vi "XCursorSlider.vi"(0 "IntensityGraph in":refnum<vi>, 1 "Cursor\nHold-off":dbl, 2 "Distance betweed scan lines (um)":sgl, 3 "Force Symmetric?":bool=TRUE) -> (4 "Scan Size X (mm)":dbl, 5 "lines per plane":i32, 6 "Scan Center (mm)":dbl)   [LabVIEW 2022 SP3]
uses:
  <vilib>/Analysis/baseanly.llb/Mean (DBL).vi
  Misc Programs/MathOperations/ModuloFraction.vi
  <vilib>/Analysis/NI_AALBase.lvlib
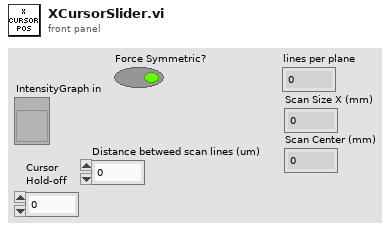
[diagram p1: front panel]
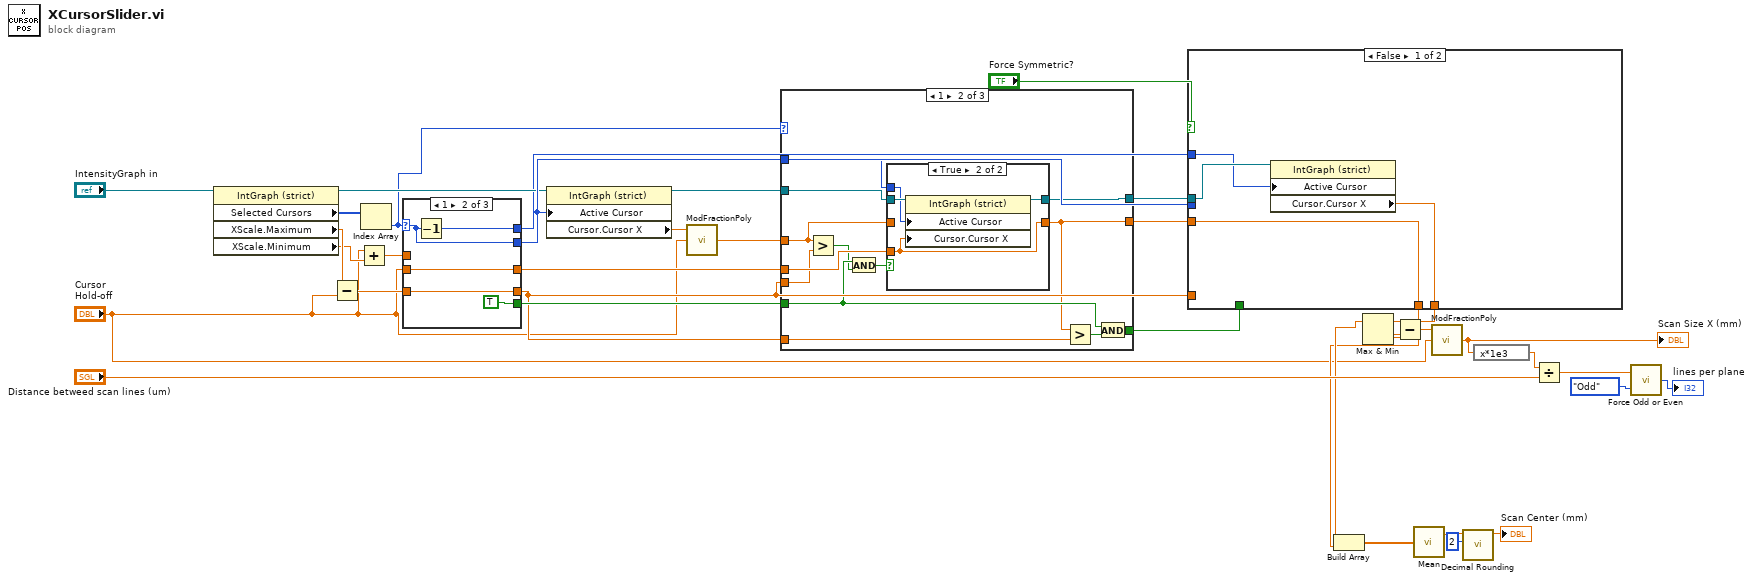
[diagram p0: block diagram]
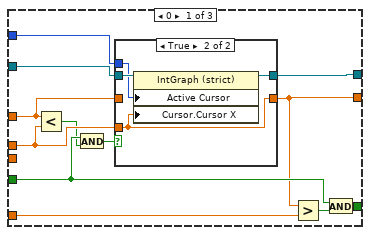
[diagram p2: hidden frame]
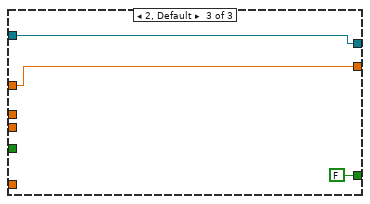
[diagram p5: hidden frame]
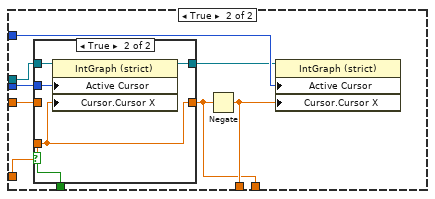
[diagram p6: hidden frame]
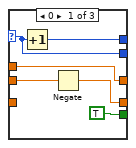
[diagram p8: hidden frame]
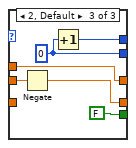
[diagram p9: hidden frame]
diagram:
  n1 = property class="IntGraph (strict)"(reference="IntensityGraph in") -> (reference out=w27:refnum<vi>, "Selected Cursors"=w25:u32[], "XScale.Maximum"=w17:dbl, "XScale.Minimum"=w16:dbl)  [unwired: 1 in, 1 out]
  n2 = Subtract(x=w17, y="Cursor\nHold-off") -> (x-y=w2:dbl)
  n3 = Add(x="Cursor\nHold-off", y=w16) -> (x+y=w29:dbl)
  n4 = Index Array(array=w25) -> (element=w4:u32)  [unwired: 1 in]
  n5 = case shown="1" w4 {
    selector: w4 -> [w38 w44 _]
    tunnel: [w38 w44 w53] -> w34
    tunnel: [TRUE TRUE FALSE] -> w33
    tunnel: [w37 w43 w51] -> w23
    tunnel: [w41 w45 w50] -> w30
    tunnel: w29 -> [w41 _ w50]
    tunnel: [w39 w46 w48] -> w3
    tunnel: w2 -> [_ w46 _]
    tunnel: "Cursor\nHold-off" -> [w40 w45 w49]
    frame 0 {
      n6 = Increment(x=w38) -> (x+1=w37:u32)
      n7 = Negate(x=w40) -> (-x=w39:dbl)
    }
    frame 1 {
      n8 = Decrement(x=w44) -> (x-1=w43:u32)
    }
    frame 2, Default {
      w53 = u32 0 ("Active Cursor")
      n9 = Negate(x=w49) -> (-x=w48:dbl)
      n10 = Increment(x=w53) -> (x+1=w51:u32)
    }
  }
  n11 = property on="Property Node" class="IntGraph (strict)"(reference=w27, "Active Cursor"=w34) -> (reference out=w28:refnum<vi>, "Cursor.Cursor X"=w35:dbl)  [unwired: 1 in, 1 out]
  n12 = call-poly "ModFractionPoly.vi"("Modulo Fraction"="Cursor\nHold-off", "Input"=w35) -> ("Output"=w36:dbl)  [unwired: 1 in]
  n13 = case shown="1" w4 {
    tunnel: w36 -> [w65 w84 w92]
    tunnel: w34 -> [w64 w83 _]
    tunnel: w33 -> [w63 w82 _]
    tunnel: [w62 w81 FALSE] -> w32
    tunnel: [w60 w79 w92] -> w31
    tunnel: w3 -> [w59 w78 _]
    tunnel: w30 -> [w58 w77 _]
    tunnel: w28 -> [w57 w76 w93]
    tunnel: [w54 w73 w93] -> w24
    tunnel: w3 -> [_ w72 _]
    frame 0 {
      n14 = Less?(x=w65, y=w58) -> (x < y?=w55:bool)
      n15 = And(x=w63, y=w55) -> (x .and. y?=w61:bool)
      n16 = case shown="True" w61 {
        tunnel: w57 -> [w66 w71]
        tunnel: w58 -> [_ w70]
        tunnel: [w67 w70] -> w60
        tunnel: w65 -> [w67 _]
        tunnel: w64 -> [_ w69]
        tunnel: [w66 w68] -> w54
        frame False {
        }
        frame True {
          n17 = property on="Property Node" class="IntGraph (strict)"(reference=w71, "Active Cursor"=w69, "Cursor.Cursor X"=w70) -> (reference out=w68:refnum<vi>)  [unwired: 1 in, 1 out]
        }
      }
      n18 = Greater?(x=w60, y=w59) -> (0:w56:bool)
      n19 = And(x=w63, y=w56) -> (x .and. y?=w62:bool)
    }
    frame 1 {
      n20 = Greater?(x=w84, y=w72) -> (0:w74:bool)
      n21 = And(x=w82, y=w74) -> (x .and. y?=w80:bool)
      n22 = case shown="True" w80 {
        tunnel: w76 -> [w85 w90]
        tunnel: w77 -> [_ w89]
        tunnel: [w86 w89] -> w79
        tunnel: w84 -> [w86 _]
        tunnel: w83 -> [_ w88]
        tunnel: [w85 w87] -> w73
        frame False {
        }
        frame True {
          n23 = property on="Property Node" class="IntGraph (strict)"(reference=w90, "Active Cursor"=w88, "Cursor.Cursor X"=w89) -> (reference out=w87:refnum<vi>)  [unwired: 1 in, 1 out]
        }
      }
      n24 = Greater?(x=w79, y=w78) -> (0:w75:bool)
      n25 = And(x=w82, y=w75) -> (x .and. y?=w81:bool)
    }
    frame 2, Default {
    }
  }
  n26 = case shown="False" "Force Symmetric?" {
    tunnel: w34 -> [_ w106]
    tunnel: w32 -> [_ w105]
    tunnel: w31 -> [w97 w104]
    tunnel: w3 -> [_ w103]
    tunnel: w24 -> [w96 w102]
    tunnel: w23 -> [w94 w101]
    tunnel: [w97 w100] -> w5
    tunnel: [w95 w98] -> w6
    frame False {
      n27 = property on="Property Node" class="IntGraph (strict)"(reference=w96, "Active Cursor"=w94) -> ("Cursor.Cursor X"=w95:dbl)  [unwired: 1 in, 2 out]
    }
    frame True {
      n28 = case shown="True" w105 {
        tunnel: w103 -> [_ w111]
        tunnel: w102 -> [w107 w112]
        tunnel: [w108 w111] -> w98
        tunnel: w104 -> [w108 _]
        tunnel: w106 -> [_ w110]
        tunnel: [w107 w109] -> w99
        frame False {
        }
        frame True {
          n29 = property on="Property Node" class="IntGraph (strict)"(reference=w112, "Active Cursor"=w110, "Cursor.Cursor X"=w111) -> (reference out=w109:refnum<vi>)  [unwired: 1 in, 1 out]
        }
      }
      n30 = Negate(x=w98) -> (-x=w100:dbl)
      n31 = property on="Property Node" class="IntGraph (strict)"(reference=w99, "Active Cursor"=w101, "Cursor.Cursor X"=w100) -> ()  [unwired: 1 in, 2 out]
    }
  }
  n32 = Build Array(w6, w5) -> (w12:dbl[])
  n33 = Max & Min(x=w6, y=w5) -> (max(x,y)=w8:dbl, min(x,y)=w7:dbl)
  n34 = Subtract(x=w8, y=w7) -> (x-y=w15:dbl)
  n35 = call-poly <vilib>:"Mean.vi"("X"=w12) -> ("mean"=w11:dbl)  [unwired: 1 out]
  n36 = call-poly "ModFractionPoly.vi"("Modulo Fraction"="Cursor\nHold-off", "Input"=w15) -> ("Output"=w14:dbl)  [unwired: 1 in]
  "Scan Size X (mm)" <- w14
  n37 = call "Decimal Rounding.vi"("Digits past \".\" (1)"=2 ("Digits past \".\" (1)"), "Input"=w11) -> ("Output"=→"Scan Center (mm)":dbl)  [unwired: 9 in]
  n38 = expression code="x*1e3"(w14) -> (w21:dbl)
  n39 = Divide(x=w21, y="Distance betweed scan lines (um)") -> (x/y=w22:dbl)
  n40 = call "Force Odd or Even.vi"("Parity (odd)"=enum16{"Odd", "Even"}."Odd" ("Parity"), "input"=w22) -> ("output"=→"lines per plane":i32)
